vi "Close.vi"(8 "error in (no error)":errorcluster, 11 "Communication in":refnum<class "Communication.lvclass">) -> (0 "error out":errorcluster)   [LabVIEW 2021, in "Communication.lvclass"]
doc: "MIT Licence\nCopyright (c) 2024 David Grollier"
uses:
  Communication.lvclass
  Communication.lvclass/Communication.ctl
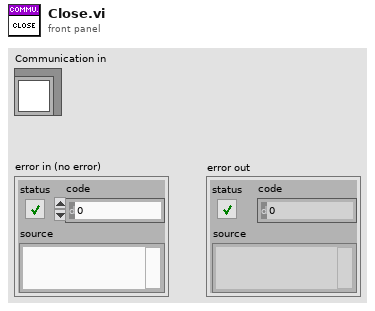
[diagram p1: front panel]
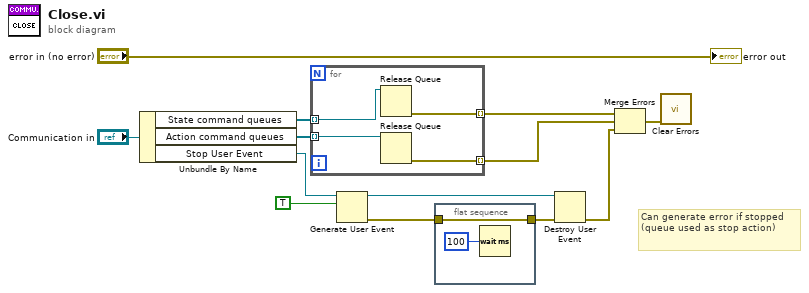
[diagram p0: block diagram]
diagram:
  # "Can generate error if stopped (queue used as stop action)"
  n1 = Unbundle By Name("Communication in") -> ("State command queues"=w12:refnum<queue>[], "Action command queues"=w10:refnum<queue>[], "Stop User Event"=w8:refnum<user-event>)
  n2 = for {
    tunnel: w12 -> [w17] mode=indexing
    tunnel: [w14] -> w11 mode=indexing
    tunnel: w10 -> [w16] mode=indexing
    tunnel: [w15] -> w9 mode=indexing
    n3 = Release Queue(queue=w17) -> (error out=w14:errorcluster)  [unwired: 2 in, 2 out]
    n4 = Release Queue(queue=w16) -> (error out=w15:errorcluster)  [unwired: 2 in, 2 out]
  }
  n5 = Generate User Event(user event=w8, event data cluster=TRUE ("event data")) -> (user event out=w6:refnum<user-event>, error out=w5:errorcluster)  [unwired: 2 in]
  n6 = flat-sequence {
    tunnel: w5 -> [w18]
    tunnel: [w18] -> w4
    frame #0 {
      n7 = Wait (ms)(milliseconds to wait=u32 100) -> ()  [unwired: 1 out]
    }
  }
  n8 = Destroy User Event(user event=w6, error in=w4) -> (error out=w3:errorcluster)
  n9 = Merge Errors(w11, w9, w3) -> (w2:errorcluster)
  n10 = call <vilib>:"Clear Errors.vi"("error in (no error)"=w2) -> ()  [unwired: 5 in, 2 out]
  "error out" <- "error in (no error)"
